vi "Constants Global.vi"() -> ()   [LabVIEW 2013]
uses:
  Constants Map typedef.ctl
  Constants typedef V2.ctl
panel:
  out "Constants Map":T1
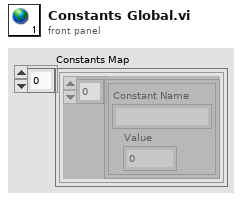
[diagram p1: front panel]
types:
  T1 = typedef "Constants Map typedef.ctl" = cluster{T2[]}[]
  T2 = typedef "Constants typedef V2.ctl" = cluster{"Constant Name":string, "Value":dbl}
diagram:
